vi "verificationSignature.vi"(2 "String":string) -> (16 "Key-ID":string, 17 "trusted":bool)   [LabVIEW 2012, in "HGF_GPG.lvlib" / "HGF_GPG.lvclass"]
doc: "called after verification. Reads the output of sysexec VI and checks whether the signing key is trusted or not"
uses:
  HGF_GPG.lvclass
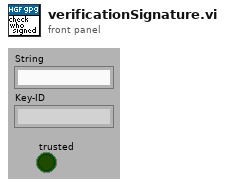
[diagram p1: front panel]
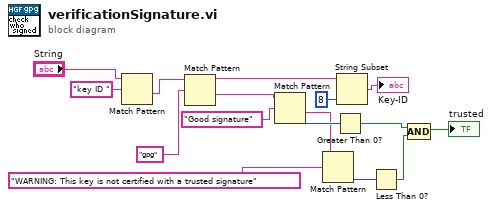
[diagram p0: block diagram]
diagram:
  n1 = Match Pattern(string="String", regular expression="key ID ") -> (after substring=w14:string)  [unwired: 4 out]
  n2 = Match Pattern(string=w14, regular expression="gpg") -> (before substring=w12:string, after substring=w8:string)  [unwired: 3 out]
  n3 = Match Pattern(string=w8, regular expression="Good signature") -> (after substring=w1:string, offset past match=w6:i32)  [unwired: 3 out]
  n4 = Match Pattern(string=w1, regular expression="WARNING: This key is not certified with a trusted signature" ("string")) -> (offset past match=w7:i32)  [unwired: 4 out]
  n5 = Greater Than 0?(x=w6) -> (x > 0?=w5:bool)
  n6 = String Subset(string=w12, length (rest)=8 ("length (rest)")) -> (substring=→"Key-ID":string)  [unwired: 1 out]
  n7 = Less Than 0?(x=w7) -> (x < 0?=w4:bool)
  n8 = Compound Arithmetic op=AND(w5, w4) -> (→"trusted":bool)
